vi "invasive_blood_pressure_measurement.vi"() -> ()   [LabVIEW 2020]
uses:
  <vilib>/Math Plots/2D Math Plots/2D Error Bar/2D Error Bar XCtrl/2D Error Bar.xctl
  <vilib>/Utility/file.llb/Write Delimited Spreadsheet (string).vi
  <vilib>/Instr/_visa.llb/VISA Configure Serial Port (Instr).vi
  <vilib>/Utility/file.llb/Write Delimited Spreadsheet (DBL).vi
  <vilib>/Math Plots/2D Math Plots/2D Error Bar/2D Error Bar Datatype/Public/Plot Helper (Fixed).vi
  <vilib>/Analysis/NI_AALBase.lvlib
  <vilib>/Math Plots/2D Math Plots/2D Error Bar/2D Error Bar Datatype/2D Error Bar Datatype.lvclass
  <vilib>/Analysis/NI_AALPro.lvlib
panel:
  out "y":i32
  in  "nule":dbl[](array[numeric])
  out "standard deviation":dbl format="%0.2f"
  out "?":T1(tab)
  in  "?":bool
  in  "baud rate (9600)":u32=9600
  in  "VISA resource name\n(izberi COM1)":refnum<visa-resource-name>
  in  "Stevilo meritev":i32
  in  "Vhodni tlaki [mmHg]":dbl[](array[numeric])
  in  "Shranjevanje podatkov":path
  in  "Cas med meritvami [s]":i32
  in  "Cas med merjenji tlaka [s]":i32
  in  "Referencni tlak [mmHg]":i32
  in  "Shranjevanje podatkov":path
  in  "Stevilo meritev":i32
  in  "Vhodna napetost [V]":i32
  in  "Vhodna napetost [V]":i32
  out "Stanje sistema":string="zacne se meritev"
  out "?":cluster{i32[], dbl[]}(graph)
  out "Povprecna vhodna napetost [V]":dbl
  out "Povprecna izhodna napetost [mV]":dbl
  in  "Prekini merjenje":bool
  out "Velikost tlaka [mmHg]":dbl(slide) scale=0.0..250.0
  out "Izmerjeni tlak [mmHg]":dbl
  out "Konec meritev":string
  out "Poteka merjenje":bool
  in  "Zacni merjenje":bool
  out "Vrednost S [qV/VmmHg]":dbl
  out "Graf vrednosti S":cluster{"napetost":dbl[], "tlak":dbl[]}(graph)
  out "Trenutni vhodni tlak [mmHg]":dbl
  out "Polnjenje tlaka":bool
  out "Zacetna vrednost premice":dbl
  out "Napaka":dbl
  out "?":cluster{i32[], dbl[]}(graph)
  out "Konec meritev":string
  in  "Ustavi merjenje":bool
  in  "Zacni merjenje":bool
  out "Poteka merjenje":bool
  out "Stanje sistema":string="zacne se meritev"
  out "Referencni tlak [mmHg]":dbl(slide) scale=0.0..250.0
  out "Izmerjeni tlak [mmHg]":dbl
  out "Povprecna izhodna napetost [mV]":dbl
  out "Izracunan povprecni\ntlak [mmHg]":dbl
  out "Korekcija tlakov":refnum<class "2D Plot Datatype.lvclass">[](xcontrol) caption="Error Bar Plot"
  in  "Izracunani tlaki [mmHg]":dbl[](array[numeric])
  out "Povprecna vhodna napetost [V]":dbl
  in  "Referencni tlak [mmHg]":dbl[](array[numeric])
  in  "Izhodne (izmerjene)\nnapetosti [mV]":dbl[](array[numeric])
  out "Izmerjeni tlaki [mmHg]":dbl[](array[numeric])
  in  "Korekcija":dbl[](array[numeric])
  out "Vrednost S [qV/VmmHg]":dbl
  in  "Standardna negotovost \nkorekcije u(K)":dbl[](array[numeric])
  # "OSNOVNE NASTAVITVE"
  # "IZVAZIVNO MERJENJE TLAKA"
  # "Invazivna metoda je metoda, ki  neposredno meri arterijski tlak. S pomocjo invazivne metode lahko preprosto belezimo dinamiko krvnega tlaka med posameznimi srcnimi utripi in dolocimo diastolicni in sistolicni krvni tlak. Invazivne metode odlikujejo najvecjo tocnost, ko jo doloca staticna in dinamicna karakteristika pretvornika tlaka."
  # "Dolocitev karakteristike sistema"
  # "Izvajanje meritev tlaka"
  # "UPORABA:\n\n1. Dolocite osnovne nastavitve\n2. Za merjenje karakteristike sistema premaknite veliki gumb levo,\n     za merjenje tlaka pa desno\n3. Vnesite zahtevane vhodne podatke\n         - Dolocitev karakteristike: \n                 * poljubno stevilo vhodnih tlakov, pri katerih se bodo    \n                    izvajale meritve\n                 * stevilo meritev, ki se izvedejo za vsak vhodni tlak\n                 * cas med posameznimi meritvami (v sekundah)\n                 * vhodna napetost, pri kateri se bodo izvajale meritve\n                 * datoteka, v katero se bodo zapisali rezultati\n         - Izvajanje meritev: \n                 * referencni tlak (za izracun merilne negotovosti)\n                 * cas med merjenji (eno merjenje obsega vec meritev, ki \n                    se izvedejo s sekundo zamika)\n                 * stevilo meritev, ki se izvedejo ob vsakem merjenju   \n                   (vsako sekundo)\n                 * vhodna napetost, pri kateri se bodo izvajale meritve\n                 * datoteka, v katero se bodo zapisali rezultati"
  # "MERJENJE TLAKOV"
  # "DOLOCITEV KARAKTERISTIKE SISTEMA"
  # "STANJE MERILNEGA SISTEMA"
  # "PODATKI NAPETOSTI"
  # "PODATKI TLAKA"
  # "REZULTAT MERJENJA KARAKTERISTIKE S"
  # "UPORABA:\n\n1.  Na zacetku SAMO ENKRAT pritisnite gumb \"Zacni \n      merjenje\". \n2.  Ce zelite z merjenjem prenehati, pritisnite gumb \n      \"Prekini merjenje\" (STOP)."
  # "STANJE MERILNEGA SISTEMA"
  # "PODATKI NAPETOSTI"
  # "PODATKI TLAKA"
  # "IZMERJENI TLAKI"
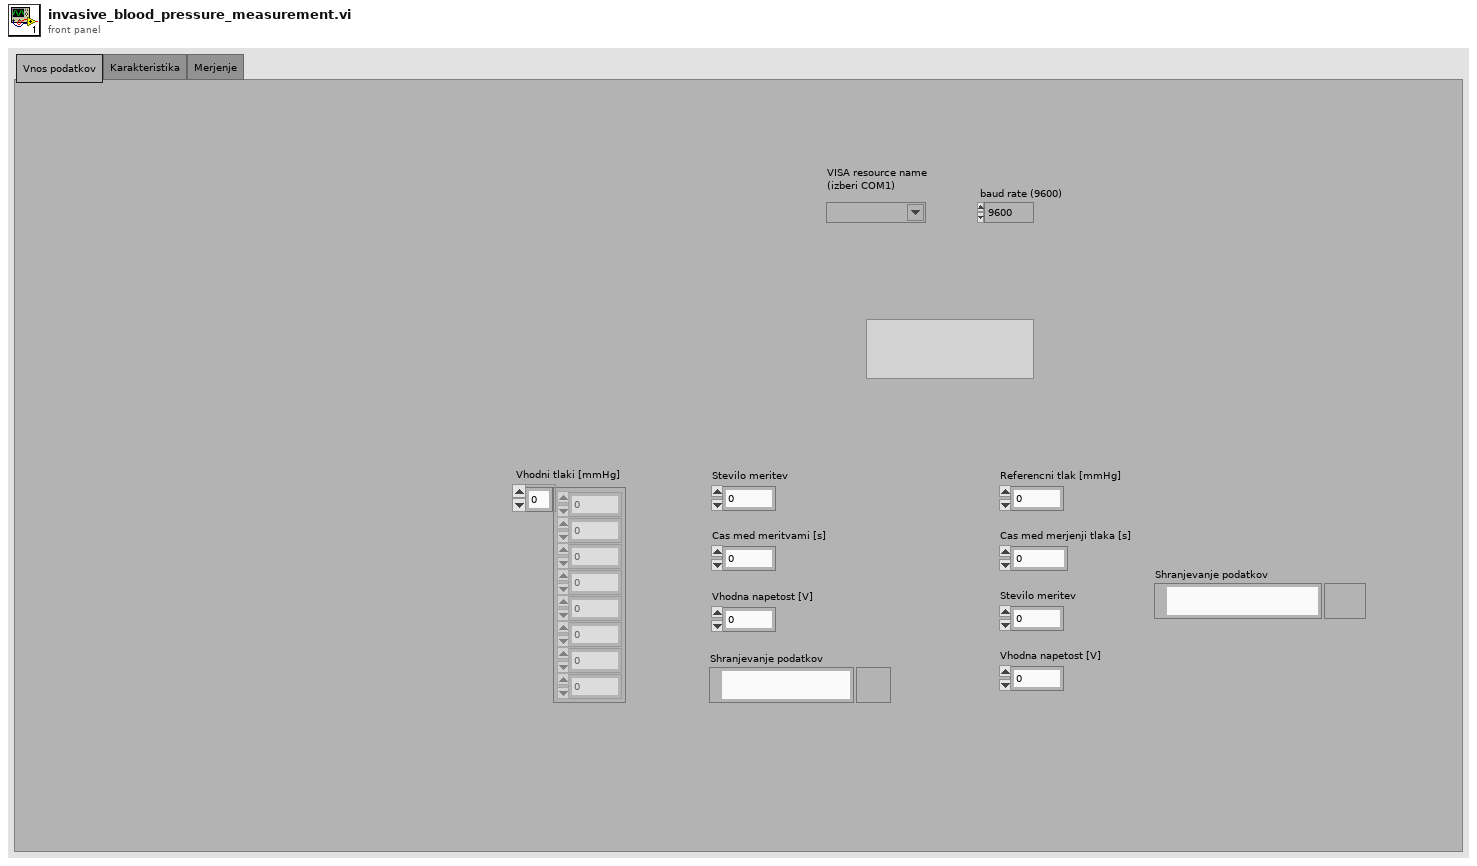
[diagram p1: front panel]
types:
  T1 = enum32{"Vnos podatkov", "Karakteristika", "Merjenje"}
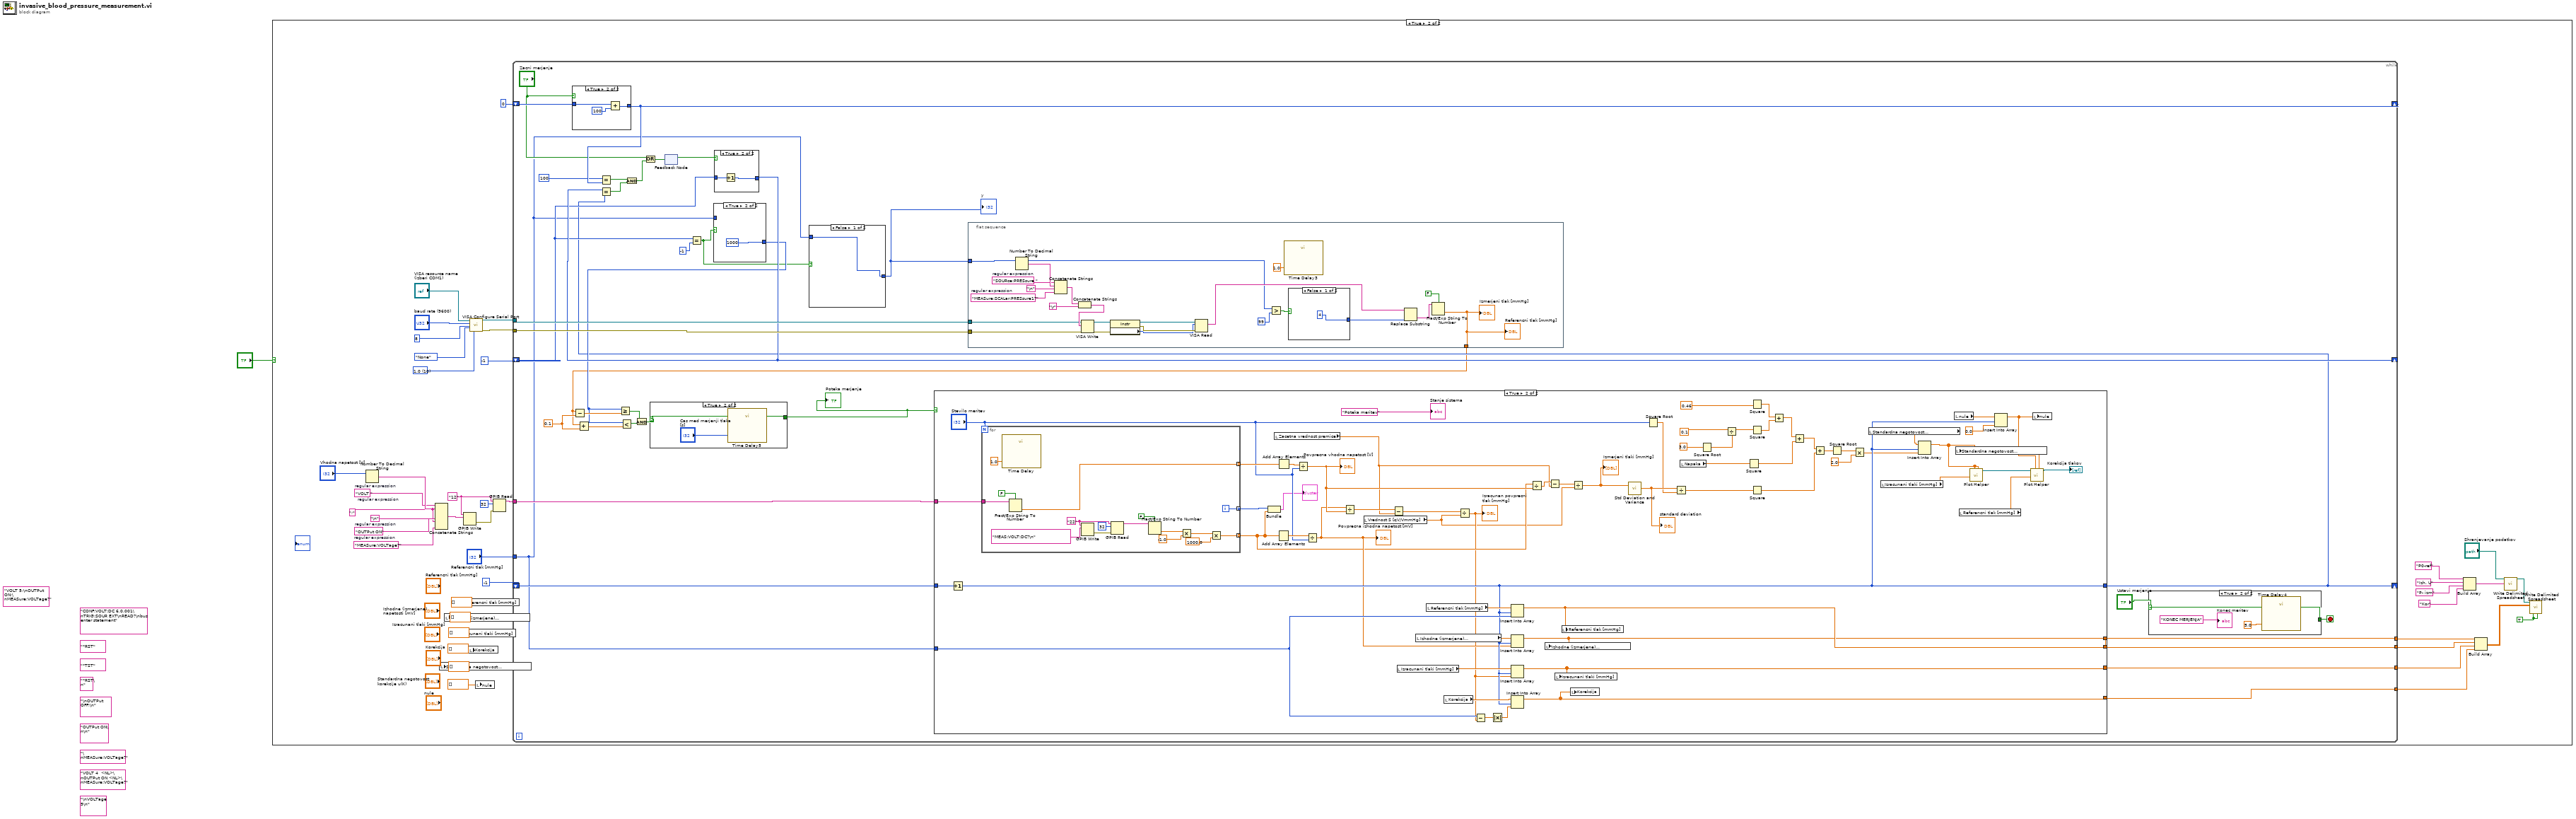
[diagram p0: block diagram]
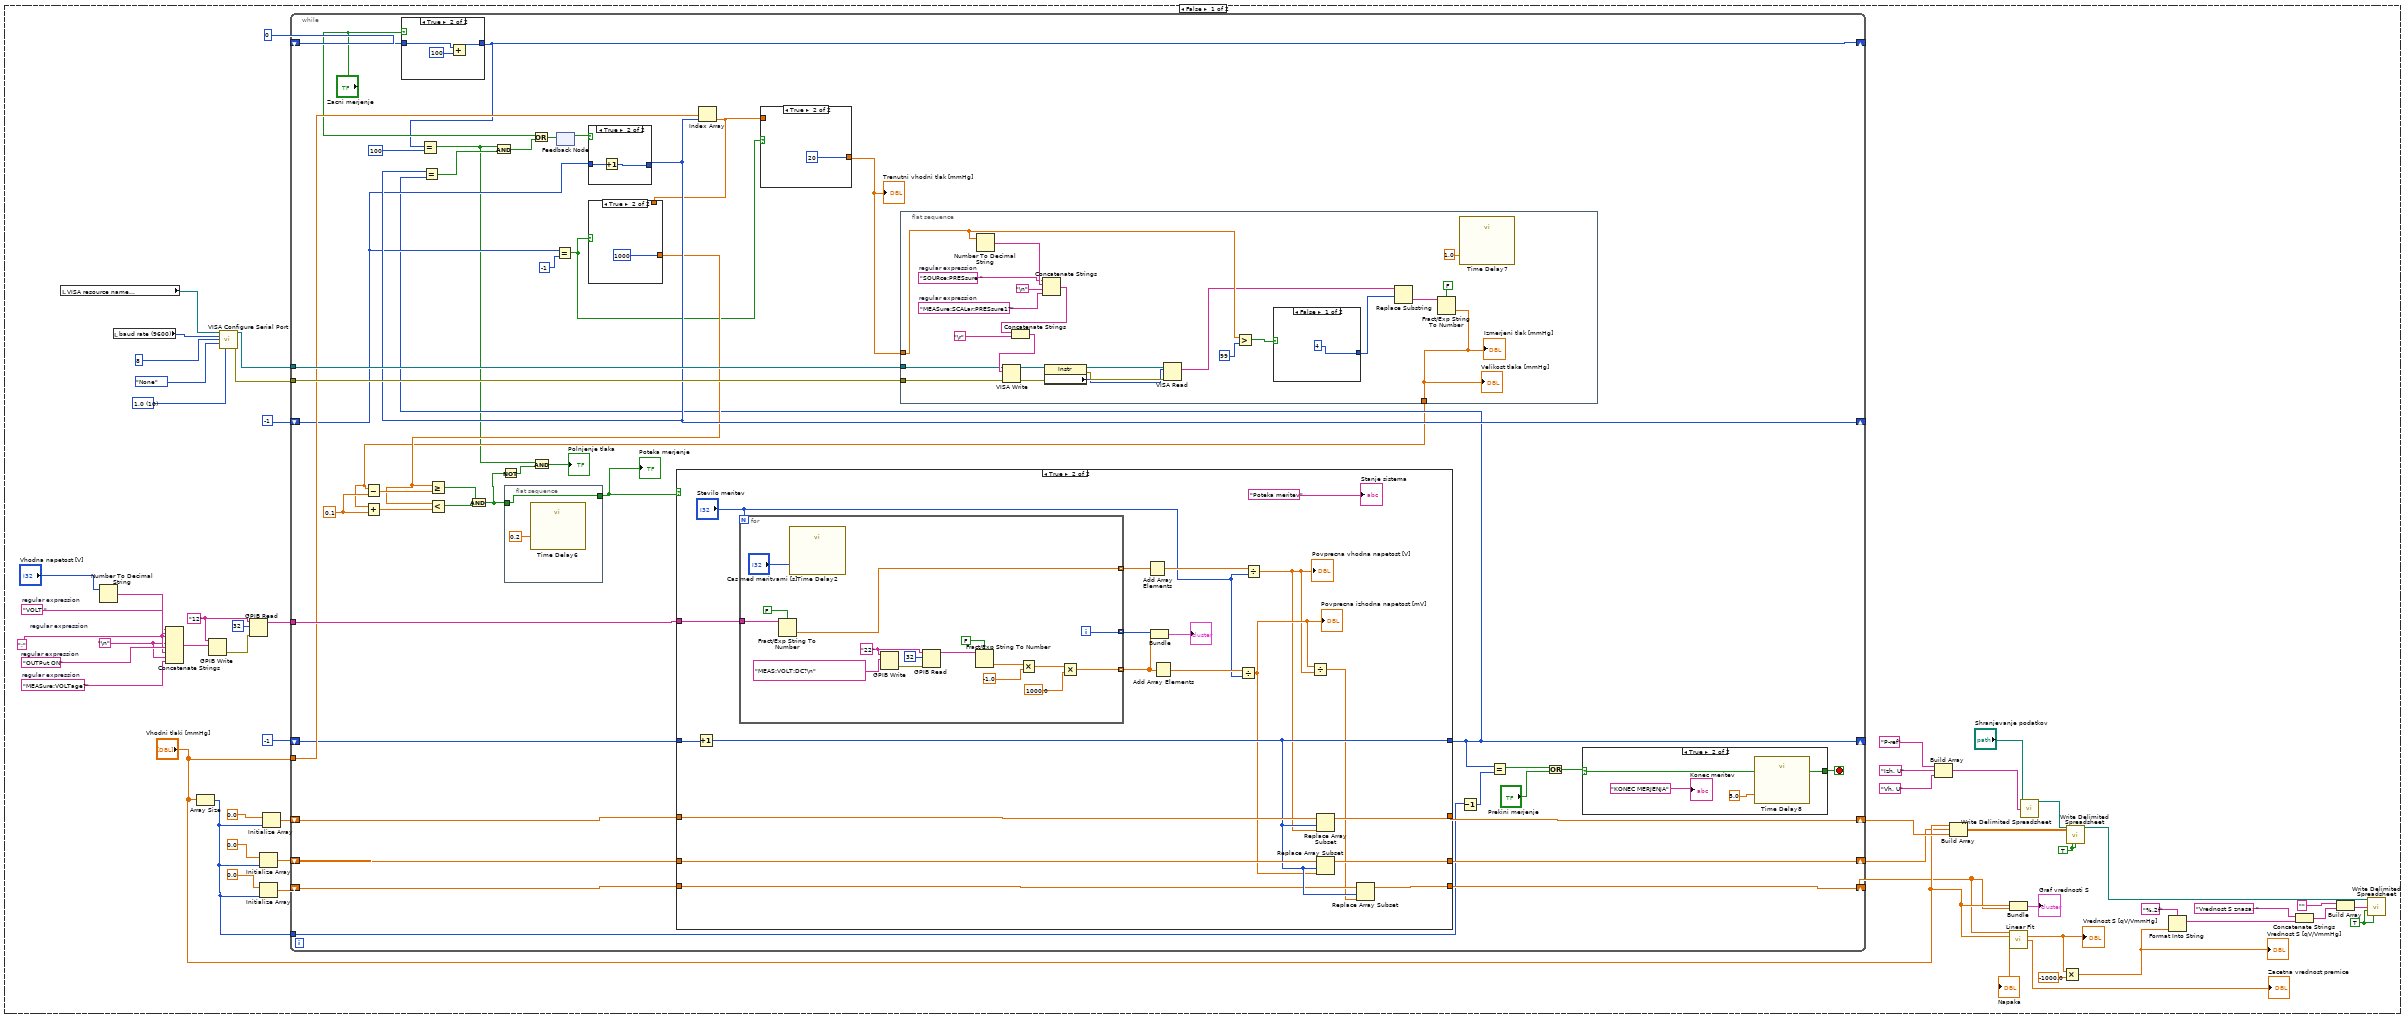
[diagram p2: hidden frame]
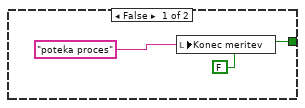
[diagram p4: hidden frame]
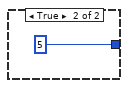
[diagram p8: hidden frame]
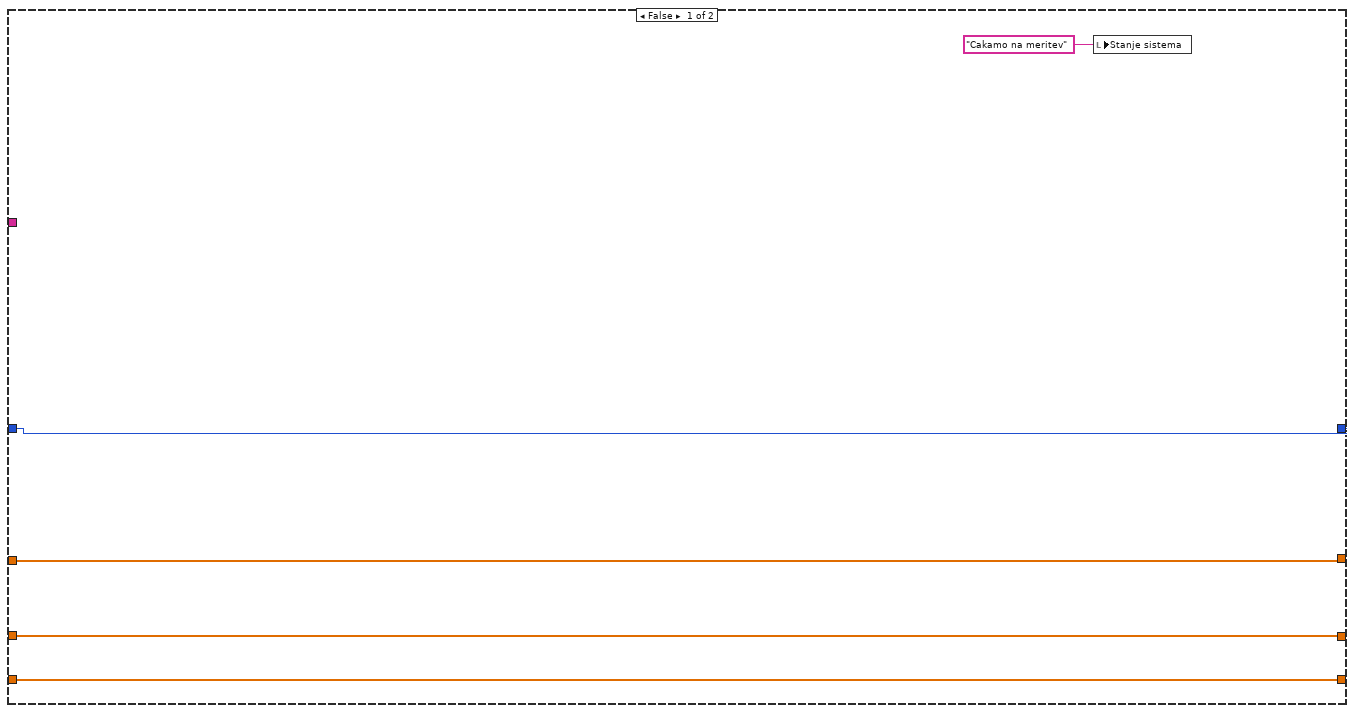
[diagram p9: hidden frame]
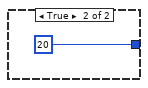
[diagram p10: hidden frame]
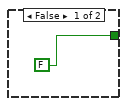
[diagram p11: hidden frame]
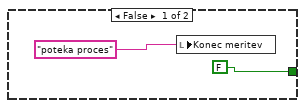
[diagram p12: hidden frame]
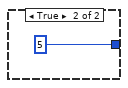
[diagram p16: hidden frame]
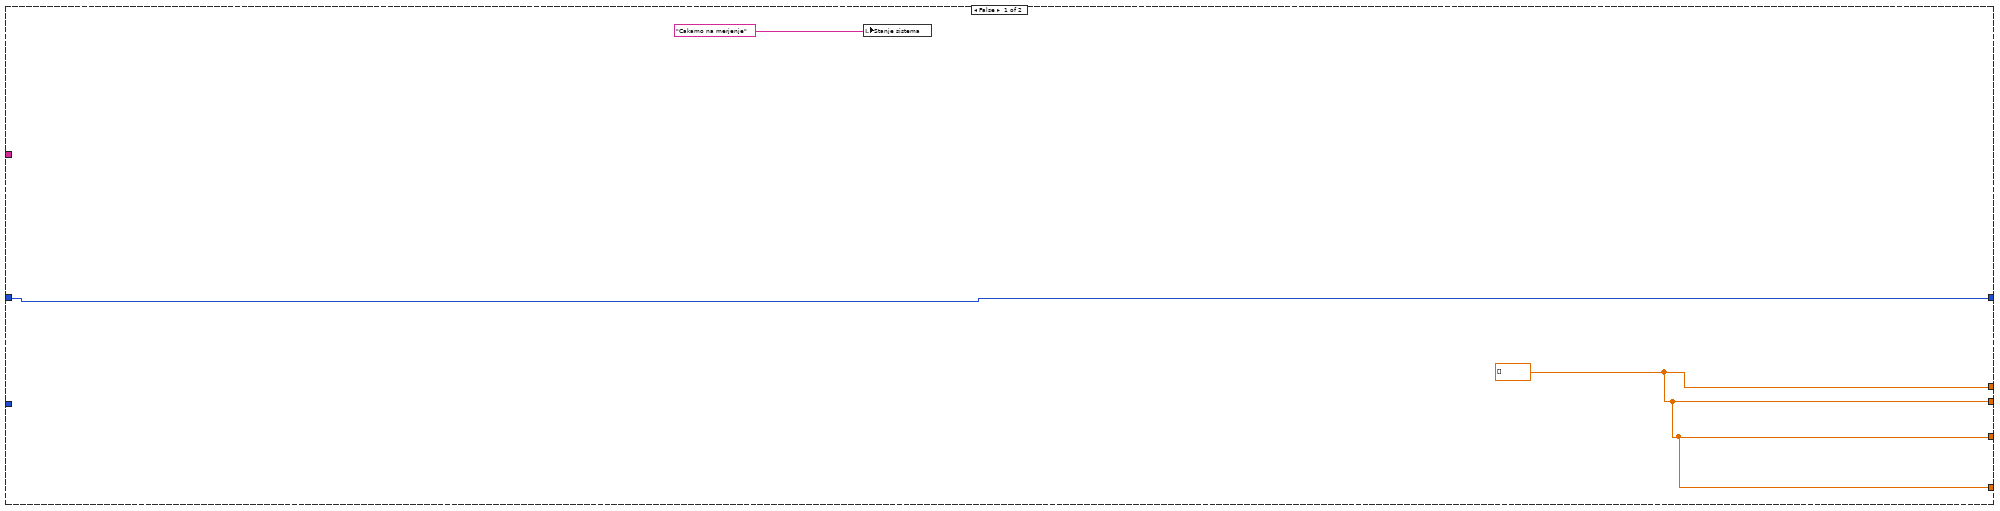
[diagram p17: hidden frame]
diagram:
  (unwired) "VOLT 5;\nOUTPut ON;\nMEASure:VOLTage?" ("data")
  (unwired) "\nOUTPut OFF;\n" ("data")
  (unwired) "\nMEASure:VOLTage?" ("data")
  (unwired) "*TST" ("data")
  (unwired) "*RST" ("data")
  (unwired) "VOLT 4  <NL>\nOUTPut ON <NL>\nMEASure:VOLTage?" ("data")
  (unwired) "\nVOLTage 5\n" ("data")
  (unwired) "*RST\n" ("data")
  (unwired) "CONF:VOLT:DC 6,0.001\nTRIG:SOUR EXT\nREAD?\nbus enter statement" ("data")
  (unwired) "OUTPut ON\n\n" ("data")
  n1 = case shown="True" "?" {
    frame False {
      w16 = u16 10 items=["1.0"=10, "1.5"=15, "2.0"=20] ("stop bits (10: 1 bit)")
      w25 = TRUE ("transpose? (no:F)")
      w32 = "MEASure:VOLTage?"  # regular expression
      w33 = "\n"
      w34 = ";"  # regular expression
      w35 = "OUTPut ON"  # regular expression
      w36 = "VOLT "  # regular expression
      w45 = TRUE ("transpose? (no:F)")
      w55 = "12" ("address string")
      n2 = local read "VISA resource name\n(izberi COM1)"() -> (w3:refnum<visa-resource-name>)
      n3 = Number To Decimal String(number="Vhodna napetost [V]") -> (decimal integer string=w37:string)  [unwired: 1 in]
      n4 = local read "baud rate (9600)"() -> (w4:u32)
      n5 = Concatenate Strings(w36, w37, w34, w33, w35, w34, w33, w32) -> (w29:string)
      n6 = Array Size(array="Vhodni tlaki [mmHg]") -> (size(s)=w11:i32)
      n7 = GPIB Write(0:w55, 1:w29) -> (6:w56:errorcluster)  [unwired: 3 in, 1 out]
      n8 = call-poly "VISA Configure Serial Port"("VISA resource name"=w3, "baud rate (9600)"=w4, "data bits (8)"=u16 8, "parity (0:none)"=enum16{"None", "Odd", "Even", "Mark", "Space"}."None", "stop bits (10: 1 bit)"=w16) -> ("VISA resource name out"=w15:refnum<visa-resource-name>, "error out"=w14:errorcluster)  [unwired: 9 in]
      n9 = GPIB Read(0:w55, 1:32 ("byte count"), 3:w56) -> (5:w53:string)  [unwired: 2 in, 2 out]
      n10 = Initialize Array(0.0 ("new element/subarray"), w11) -> (w40:dbl[])
      n11 = Initialize Array(0.0 ("new element/subarray"), w11) -> (w30:dbl[])
      n12 = Initialize Array(0.0 ("new element/subarray"), w11) -> (w50:dbl[])
      n13 = while {
        tunnel: w53 -> [w100]
        tunnel: "Vhodni tlaki [mmHg]" -> [w90]
        shift-right: [w74] -> _
        shift-left: -1 -> [w81]
        shift-right: [w98] -> w39
        shift-left: w50 -> [w95]
        shift-right: [w97] -> w27
        shift-left: w40 -> [w96]
        shift-right: [w93] -> w19
        shift-left: w30 -> [w94]
        tunnel: w15 -> [w92]
        tunnel: w14 -> [w91]
        shift-right: [w80] -> _
        shift-left: -1 -> [w76]
        shift-right: [w58] -> _
        shift-left: 0 -> [w85]
        tunnel: w11 -> [w73]
        stop <- w68 stop-if-true
        w89 = 0.1 ("y")
        n14 = Subtract(x=w67, y=w89) -> (x-y=w87:dbl)
        n15 = Add(x=w67, y=w89) -> (x+y=w88:dbl)
        n16 = case shown="True" "Zacni merjenje" {
          tunnel: w85 -> [w110 w113]
          tunnel: [w110 w111] -> w58
          frame False {
          }
          frame True {
            n17 = Add(x=w113, y=100) -> (x+y=w111:i32)
          }
        }
        n18 = Equal?(x=w58, y=100 ("x")) -> (x = y?=w62:bool)
        n19 = flat-sequence {
          tunnel: w61 -> [w142]
          tunnel: [w142] -> w99
          frame #0 {
            n20 = call "Time Delay6"("Delay Time (s)"=0.2) -> ()  [unwired: 10 in, 1 out]
          }
        }
        n21 = Equal?(x=w76, y=-1) -> (x = y?=w66:bool)
        n22 = feedback #1() -> (w82:bool)  [unwired: 1 in]
        n23 = case shown="True" w82 {
          tunnel: w76 -> [w114 w116]
          tunnel: [w114 w115] -> w80
          frame False {
          }
          frame True {
            n24 = Increment(x=w116) -> (x+1=w115:i32)
          }
        }
        n25 = case shown="True" w99 {
          tunnel: w100 -> [_ w161]
          tunnel: [w144 w160] -> w98
          tunnel: [w147 w159] -> w97
          tunnel: w96 -> [w147 w158]
          tunnel: w95 -> [w144 w157]
          tunnel: w81 -> [w148 w156]
          tunnel: [w148 w154] -> w74
          tunnel: w94 -> [w145 w153]
          tunnel: [w145 w152] -> w93
          frame False {
            n26 = local write "Stanje sistema"("Cakamo na meritev") -> ()
          }
          frame True {
            n27 = Increment(x=w156) -> (x+1=w154:i32)
            n28 = for {
              N: "Stevilo meritev" -> [_]
              tunnel: [w173] -> w163 mode=indexing
              tunnel: [w172] -> w167 mode=indexing
              tunnel: [w171] -> w164 mode=indexing
              tunnel: w161 -> [w170]
              i -> [w171]
              w184 = "22" ("address string")
              n29 = Fract/Exp String To Number(use system decimal point (T)=FALSE, string=w170) -> (number=w172:dbl)  [unwired: 2 in, 1 out]
              n30 = call "Time Delay2"("Delay Time (s)"="Cas med meritvami [s]") -> ()  [unwired: 10 in, 1 out]
              n31 = GPIB Write(0:w184, 1:"MEAS:VOLT:DC?\n" ("data")) -> (6:w182:errorcluster)  [unwired: 3 in, 1 out]
              n32 = GPIB Read(0:w184, 1:32 ("byte count"), 3:w182) -> (5:w176:string)  [unwired: 2 in, 2 out]
              n33 = Fract/Exp String To Number(use system decimal point (T)=FALSE, string=w176) -> (number=w180:dbl)  [unwired: 2 in, 1 out]
              n34 = Multiply(x=w180, y=-1.0) -> (x*y=w175:dbl)
              n35 = Multiply(x=w175, y=1000.0) -> (x*y=w173:dbl)
            }
            n36 = Add Array Elements(numeric array=w167) -> (sum=w166:dbl)
            n37 = Bundle(w164, w163) -> (→"?":cluster{i32[], dbl[]})  [unwired: 1 in]
            n38 = Add Array Elements(numeric array=w163) -> (sum=w168:dbl)
            n39 = Divide(x=w168, y="Stevilo meritev") -> (x/y=w151:dbl)
            "Povprecna izhodna napetost [mV]" <- w151
            n40 = Divide(x=w166, y="Stevilo meritev") -> (x/y=w150:dbl)
            "Povprecna vhodna napetost [V]" <- w150
            n41 = Divide(x=w151, y=w150) -> (x/y=w149:dbl)
            n42 = Replace Array Subset(array=w157, new element=w150, index=w154) -> (w160:dbl[])
            n43 = Replace Array Subset(array=w158, new element=w151, index=w154) -> (w159:dbl[])
            n44 = Replace Array Subset(array=w153, new element=w149, index=w154) -> (w152:dbl[])
            "Stanje sistema" <- "Poteka meritev"
          }
        }
        n45 = Equal?(x=w80, y=w74) -> (x = y?=w79:bool)
        n46 = And(x=w62, y=w79) -> (x .and. y?=w78:bool)
        n47 = Or(x="Zacni merjenje", y=w78) -> (x .or. y?=w83:bool)
        n48 = feedback-in #1(w83) -> ()
        n49 = Index Array(array=w90, index=w80) -> (element=w64:dbl)
        n50 = case shown="True" w66 {
          tunnel: [w108 1000 ("y")] -> w75
          tunnel: w64 -> [w108 _]
          frame False {
          }
          frame True {
          }
        }
        n51 = Greater Or Equal?(x=w75, y=w87) -> (x >= y?=w63:bool)
        n52 = Less?(x=w75, y=w88) -> (x < y?=w86:bool)
        n53 = And(x=w63, y=w86) -> (x .and. y?=w61:bool)
        n54 = Not(x=w61) -> (.not. x?=w60:bool)
        n55 = And(x=w62, y=w60) -> (x .and. y?=→"Polnjenje tlaka":bool)
        n56 = case shown="True" w66 {
          tunnel: [w101 20 ("y")] -> w65
          tunnel: w64 -> [w101 _]
          frame False {
          }
          frame True {
          }
        }
        "Trenutni vhodni tlak [mmHg]" <- w65
        n57 = flat-sequence {
          tunnel: w92 -> [w127]
          tunnel: w91 -> [w126]
          tunnel: w65 -> [w119]
          tunnel: [w117] -> w67
          frame #0 {
            w129 = "MEASure:SCALar:PRESsure1?"  # regular expression
            w131 = "SOURce:PRESsure "  # regular expression
            n58 = Number To Decimal String(number=w119) -> (decimal integer string=w132:string)  [unwired: 1 in]
            n59 = Concatenate Strings(w131, w132, "\n", w129) -> (w128:string)
            n60 = Concatenate Strings(w128, "\r") -> (w133:string)
            n61 = VISA Write(VISA resource name=w127, write buffer=w133, error in (no error)=w126) -> (VISA resource name out=w139:refnum<visa-resource-name>, error out=w136:errorcluster)  [unwired: 1 out]
            n62 = property class="Instr"(reference=w139, error in=w136) -> (reference out=w138:refnum<visa-resource-name>, error out=w137:errorcluster, "Serial Settings:Number of Bytes at Serial Port"=w135:u32)
            n63 = VISA Read(VISA resource name=w138, byte count=w135, error in (no error)=w137) -> (read buffer=w118:string)  [unwired: 3 out]
            n64 = Greater?(x=w119, y=99) -> (0:w123:bool)
            n65 = case shown="False" w123 {
              tunnel: [4 ("y") 5 ("y")] -> w122
              frame False {
              }
              frame True {
              }
            }
            n66 = Replace Substring(2:w122, 5:w118) -> (0:w121:string)  [unwired: 2 in, 1 out]
            n67 = Fract/Exp String To Number(use system decimal point (T)=FALSE, string=w121) -> (number=w117:dbl)  [unwired: 2 in, 1 out]
            "Izmerjeni tlak [mmHg]" <- w117
            "Velikost tlaka [mmHg]" <- w117
            n68 = call "Time Delay7"("Delay Time (s)"=1.0) -> ()  [unwired: 10 in, 1 out]
          }
        }
        n69 = Decrement(x=w73) -> (x-1=w72:i32)
        n70 = Equal?(x=w74, y=w72) -> (x = y?=w70:bool)
        n71 = Or(x=w70, y="Prekini merjenje") -> (x .or. y?=w69:bool)
        n72 = case shown="True" w69 {
          selector: w69 -> [_ w105]
          tunnel: [FALSE w105] -> w68
          frame False {
            n73 = local write "Konec meritev"("poteka proces") -> ()
          }
          frame True {
            n74 = call "Time Delay8"("Delay Time (s)"=5.0) -> ()  [unwired: 10 in, 1 out]
            "Konec meritev" <- "KONEC MERJENJA"
          }
        }
        "Poteka merjenje" <- w99
      }
      n75 = Build Array("P-ref", "Izh. U", "Vh. U") -> (w47:string[])
      n76 = Build Array("Vhodni tlaki [mmHg]", w27, w39) -> (w43:dbl[][])
      n77 = Bundle("Vhodni tlaki [mmHg]"="Vhodni tlaki [mmHg]", w19) -> (→"Graf vrednosti S":cluster{" Vhodni tlaki [mmHg]":dbl[], dbl[]})  [unwired: 1 in]
      n78 = call <vilib>:"Linear Fit.vi"("Y"=w19, "X"="Vhodni tlaki [mmHg]") -> ("slope"=w8:dbl, "intercept"=→"Zacetna vrednost premice":dbl, "residue"=→"Napaka":dbl)  [unwired: 9 in, 2 out]
      "Vrednost S [qV/VmmHg]" <- w8
      n79 = call-poly <vilib>:"Write Delimited Spreadsheet.vi"("file path (dialog if empty)"="Shranjevanje podatkov", "1D data"=w47) -> ("new file path (Not A Path if cancelled)"=w46:path)  [unwired: 12 in, 1 out]
      n80 = Multiply(x=w8, y=-1000.0) -> (x*y=w6:dbl)
      "Vrednost S [qV/VmmHg]" <- w6
      n81 = call-poly <vilib>:"Write Delimited Spreadsheet.vi"("file path (dialog if empty)"=w46, "2D data"=w43, "append to file? (new file:F)"=w45, "transpose? (no:F)"=w45) -> ("new file path (Not A Path if cancelled)"=w20:path)  [unwired: 10 in, 1 out]
      n82 = Format Into String(format string="%.2f", w6) -> (resulting string=w7:string)  [unwired: 2 in, 1 out]
      n83 = Concatenate Strings("Vrednost S znasa: ", w7) -> (w21:string)
      n84 = Build Array("", w21) -> (w24:string[])
      n85 = call-poly <vilib>:"Write Delimited Spreadsheet.vi"("file path (dialog if empty)"=w20, "1D data"=w24, "append to file? (new file:F)"=w25, "transpose? (no:F)"=w25) -> ()  [unwired: 10 in, 2 out]
    }
    frame True {
      w202 = u16 10 items=["1.0"=10, "1.5"=15, "2.0"=20] ("stop bits (10: 1 bit)")
      w208 = "MEASure:VOLTage?"  # regular expression
      w209 = "\n"
      w210 = ";"  # regular expression
      w211 = "OUTPut ON"  # regular expression
      w212 = "VOLT "  # regular expression
      w217 = TRUE ("transpose? (no:F)")
      w225 = "12" ("address string")
      n86 = Number To Decimal String(number="Vhodna napetost [V]") -> (decimal integer string=w213:string)  [unwired: 1 in]
      n87 = Concatenate Strings(w212, w213, w210, w209, w211, w210, w209, w208) -> (w207:string)
      n88 = local write "Standardna negotovost \nkorekcije u(K)"(dbl[] []) -> ()
      n89 = local write "Izhodne (izmerjene)\nnapetosti [mV]"(dbl[] []) -> ()
      n90 = local write "Izracunani tlaki [mmHg]"(dbl[] []) -> ()
      n91 = local write "Referencni tlak [mmHg]"(dbl[] []) -> ()
      n92 = GPIB Write(0:w225, 1:w207) -> (6:w226:errorcluster)  [unwired: 3 in, 1 out]
      n93 = local write "Korekcija"(dbl[] []) -> ()
      n94 = call-poly "VISA Configure Serial Port"("VISA resource name"="VISA resource name\n(izberi COM1)", "baud rate (9600)"="baud rate (9600)", "data bits (8)"=u16 8, "parity (0:none)"=enum16{"None", "Odd", "Even", "Mark", "Space"}."None", "stop bits (10: 1 bit)"=w202) -> ("VISA resource name out"=w201:refnum<visa-resource-name>, "error out"=w200:errorcluster)  [unwired: 9 in]
      n95 = local write "nule"(dbl[] []) -> ()
      n96 = GPIB Read(0:w225, 1:32 ("byte count"), 3:w226) -> (5:w223:string)  [unwired: 2 in, 2 out]
      n97 = while {
        tunnel: w223 -> [w261]
        shift-right: [w240] -> _
        shift-left: -1 -> [w248]
        tunnel: w201 -> [w260]
        tunnel: w200 -> [w259]
        shift-right: [w246] -> _
        shift-left: -1 -> [w242]
        shift-right: [w253] -> _
        shift-left: 0 -> [w254]
        tunnel: "Referencni tlak [mmHg]" -> [w234]
        tunnel: [w230] -> w188
        tunnel: [w229] -> w187
        tunnel: [w228] -> w186
        tunnel: [w227] -> w185
        stop <- w239 stop-if-true
        w238 = 0.1 ("y")
        n98 = case shown="True" "Zacni merjenje" {
          tunnel: w254 -> [w274 w277]
          tunnel: [w274 w275] -> w253
          frame False {
          }
          frame True {
            n99 = Add(x=w277, y=100) -> (x+y=w275:i32)
          }
        }
        n100 = Subtract(x=w235, y=w238) -> (x-y=w257:dbl)
        n101 = Add(x=w235, y=w238) -> (x+y=w258:dbl)
        n102 = Equal?(x=100, y=w253) -> (x = y?=w247:bool)
        n103 = feedback #2() -> (w249:bool)  [unwired: 1 in]
        n104 = Equal?(x=w242, y=-1) -> (x = y?=w232:bool)
        n105 = case shown="True" w232 {
          tunnel: [w272 1000 ("y")] -> w241
          tunnel: w234 -> [w272 _]
          frame False {
          }
          frame True {
          }
        }
        n106 = Greater Or Equal?(x=w241, y=w257) -> (x >= y?=w256:bool)
        n107 = Less?(x=w241, y=w258) -> (x < y?=w255:bool)
        n108 = And(x=w256, y=w255) -> (x .and. y?=w237:bool)
        n109 = case shown="True" w237 {
          selector: w237 -> [_ w266]
          tunnel: [FALSE w266] -> w231
          frame False {
          }
          frame True {
            n110 = call "Time Delay5"("Delay Time (s)"="Cas med merjenji tlaka [s]") -> ()  [unwired: 10 in, 1 out]
          }
        }
        "Poteka merjenje" <- w231
        n111 = case shown="True" w249 {
          tunnel: w242 -> [w278 w280]
          tunnel: [w278 w279] -> w246
          frame False {
          }
          frame True {
            n112 = Increment(x=w280) -> (x+1=w279:i32)
          }
        }
        n113 = case shown="False" w232 {
          tunnel: [w262 20 ("y")] -> w233
          tunnel: w234 -> [w262 _]
          frame False {
          }
          frame True {
          }
        }
        "y" <- w233
        n114 = case shown="True" w231 {
          tunnel: w261 -> [_ w364]
          tunnel: w248 -> [w308 w363]
          tunnel: [w308 w340] -> w240
          tunnel: w234 -> [_ w347]
          tunnel: [w306 w339] -> w230
          tunnel: [w306 w338] -> w229
          tunnel: [w306 w337] -> w228
          tunnel: [w306 w336] -> w227
          frame False {
            w306 = dbl[] []
            n115 = local write "Stanje sistema"("Cakamo na merjenje") -> ()
          }
          frame True {
            n116 = Increment(x=w363) -> (x+1=w340:i32)
            n117 = for {
              N: "Stevilo meritev" -> [_]
              tunnel: [w372] -> w319 mode=indexing
              tunnel: [w371] -> w367 mode=indexing
              tunnel: [w370] -> w365 mode=indexing
              tunnel: w364 -> [w369]
              i -> [w370]
              w384 = "22" ("address string")
              n118 = call "Time Delay"("Delay Time (s)"=1.0) -> ()  [unwired: 10 in, 1 out]
              n119 = Fract/Exp String To Number(use system decimal point (T)=FALSE, string=w369) -> (number=w371:dbl)  [unwired: 2 in, 1 out]
              n120 = GPIB Write(0:w384, 1:"MEAS:VOLT:DC?\n" ("data")) -> (6:w382:errorcluster)  [unwired: 3 in, 1 out]
              n121 = GPIB Read(0:w384, 1:32 ("byte count"), 3:w382) -> (5:w375:string)  [unwired: 2 in, 2 out]
              n122 = Fract/Exp String To Number(use system decimal point (T)=FALSE, string=w375) -> (number=w379:dbl)  [unwired: 2 in, 1 out]
              n123 = Multiply(x=w379, y=-1.0) -> (x*y=w374:dbl)
              n124 = Multiply(x=w374, y=1000.0) -> (x*y=w372:dbl)
            }
            n125 = Bundle(w365, w319) -> (→"?":cluster{i32[], dbl[]})  [unwired: 1 in]
            n126 = local read "Zacetna vrednost premice"() -> (w311:dbl)
            n127 = Add Array Elements(numeric array=w319) -> (sum=w368:dbl)
            n128 = Add Array Elements(numeric array=w367) -> (sum=w366:dbl)
            n129 = Divide(x=w366, y="Stevilo meritev") -> (x/y=w352:dbl)
            "Povprecna vhodna napetost [V]" <- w352
            n130 = Divide(x=w368, y="Stevilo meritev") -> (x/y=w320:dbl)
            "Povprecna izhodna napetost [mV]" <- w320
            n131 = Divide(x=w320, y=w352) -> (x/y=w313:dbl)
            n132 = local read "Vrednost S [qV/VmmHg]"() -> (w315:dbl)
            n133 = Subtract(x=w313, y=w311) -> (x-y=w318:dbl)
            n134 = local read "Izracunani tlaki [mmHg]"() -> (w349:dbl[])
            n135 = local read "Izhodne (izmerjene)\nnapetosti [mV]"() -> (w346:dbl[])
            n136 = local read "Referencni tlak [mmHg]"() -> (w348:dbl[])
            n137 = local read "Korekcija"() -> (w351:dbl[])
            n138 = Divide(x=w318, y=w315) -> (x/y=w317:dbl)
            "Izracunan povprecni\ntlak [mmHg]" <- w317
            n139 = Subtract(x=w347, y=w317) -> (x-y=w361:dbl)
            n140 = Absolute Value(x=w361) -> (abs(x)=w350:dbl)
            n141 = Insert Into Array(array=w348, index=w340, new element=w347) -> (w339:dbl[])
            n142 = Insert Into Array(array=w346, index=w340, new element=w320) -> (w338:dbl[])
            n143 = Insert Into Array(array=w349, index=w340, new element=w317) -> (w337:dbl[])
            n144 = Insert Into Array(array=w351, index=w340, new element=w350) -> (w336:dbl[])
            n145 = Divide(x=w319, y=w352) -> (x/y=w312:dbl[])
            n146 = local write "Izhodne (izmerjene)\nnapetosti [mV]"(w338) -> ()
            n147 = Subtract(x=w312, y=w311) -> (x-y=w316:dbl[])
            n148 = local write "Izracunani tlaki [mmHg]"(w337) -> ()
            n149 = local write "Referencni tlak [mmHg]"(w339) -> ()
            n150 = local write "Korekcija"(w336) -> ()
            n151 = Divide(x=w316, y=w315) -> (x/y=w314:dbl[])
            "Izmerjeni tlaki [mmHg]" <- w314
            n152 = call <vilib>:"Std Deviation and Variance.vi"("X"=w314) -> ("standard deviation"=w359:dbl)  [unwired: 1 in, 2 out]
            "standard deviation" <- w359
            n153 = Square Root(x="Stevilo meritev") -> (sqrt(x)=w358:dbl)
            n154 = Divide(x=w359, y=w358) -> (x/y=w327:dbl)
            n155 = local read "Napaka"() -> (w309:dbl)
            n156 = Square Root(x=3.0) -> (sqrt(x)=w331:dbl)
            n157 = Divide(x=0.1, y=w331) -> (x/y=w329:dbl)
            n158 = Square(x=w309) -> (x^2=w333:dbl)
            n159 = Square(x=0.46) -> (x^2=w335:dbl)
            n160 = Square(x=w329) -> (x^2=w332:dbl)
            n161 = Square(x=w327) -> (x^2=w326:dbl)
            n162 = Add(x=w335, y=w332) -> (x+y=w334:dbl)
            n163 = Add(x=w334, y=w333) -> (x+y=w325:dbl)
            n164 = Add(x=w325, y=w326) -> (x+y=w324:dbl)
            n165 = Square Root(x=w324) -> (sqrt(x)=w322:dbl)
            n166 = Multiply(x=w322, y=2.0) -> (x*y=w321:dbl)
            n167 = local read "Standardna negotovost \nkorekcije u(K)"() -> (w342:dbl[])
            n168 = local read "Izracunani tlaki [mmHg]"() -> (w357:dbl[])
            n169 = Insert Into Array(array=w342, index=w340, new element=w321) -> (w341:dbl[])
            n170 = local read "nule"() -> (w344:dbl[])
            n171 = local write "Standardna negotovost \nkorekcije u(K)"(w341) -> ()
            n172 = local read "Referencni tlak [mmHg]"() -> (w354:dbl[])
            n173 = call-poly <vilib>:"Plot Helper.vi"("error b vector"=w341, "error a vector"=w341, "y vector"=w357) -> ("2D Plot Class Obj Array out"=w356:refnum<class "2D Plot Datatype.lvclass">[])  [unwired: 3 in, 5 out]
            n174 = Insert Into Array(array=w344, index=w340, new element=0.0 ("new element/subarray")) -> (w343:dbl[])
            n175 = call-poly <vilib>:"Plot Helper.vi"("error b vector"=w343, "error a vector"=w343, "y vector"=w354, "2D Plot Class Obj Array in"=w356) -> ("2D Plot Class Obj Array out"=→"Korekcija tlakov":refnum<class "2D Plot Datatype.lvclass">[])  [unwired: 2 in, 5 out]
            n176 = local write "nule"(w343) -> ()
            "Stanje sistema" <- "Poteka meritev"
          }
        }
        n177 = Equal?(x=w246, y=w240) -> (x = y?=w245:bool)
        n178 = And(x=w247, y=w245) -> (x .and. y?=w244:bool)
        n179 = Or(x="Zacni merjenje", y=w244) -> (x .or. y?=w250:bool)
        n180 = feedback-in #2(w250) -> ()
        n181 = flat-sequence {
          tunnel: w260 -> [w291]
          tunnel: w259 -> [w290]
          tunnel: w233 -> [w281]
          tunnel: [w282] -> w235
          frame #0 {
            w293 = "MEASure:SCALar:PRESsure1?"  # regular expression
            w295 = "SOURce:PRESsure "  # regular expression
            n182 = Number To Decimal String(number=w281) -> (decimal integer string=w296:string)  [unwired: 1 in]
            n183 = Concatenate Strings(w295, w296, "\n", w293) -> (w292:string)
            n184 = Concatenate Strings(w292, "\r") -> (w297:string)
            n185 = VISA Write(VISA resource name=w291, write buffer=w297, error in (no error)=w290) -> (VISA resource name out=w303:refnum<visa-resource-name>, error out=w300:errorcluster)  [unwired: 1 out]
            n186 = property class="Instr"(reference=w303, error in=w300) -> (reference out=w302:refnum<visa-resource-name>, error out=w301:errorcluster, "Serial Settings:Number of Bytes at Serial Port"=w299:u32)
            n187 = VISA Read(VISA resource name=w302, byte count=w299, error in (no error)=w301) -> (read buffer=w283:string)  [unwired: 3 out]
            n188 = Greater?(x=w281, y=99) -> (0:w287:bool)
            n189 = call "Time Delay3"("Delay Time (s)"=1.0) -> ()  [unwired: 10 in, 1 out]
            n190 = case shown="False" w287 {
              tunnel: [4 ("y") 5 ("y")] -> w286
              frame False {
              }
              frame True {
              }
            }
            n191 = Replace Substring(2:w286, 5:w283) -> (0:w285:string)  [unwired: 2 in, 1 out]
            n192 = Fract/Exp String To Number(use system decimal point (T)=FALSE, string=w285) -> (number=w282:dbl)  [unwired: 2 in, 1 out]
            "Izmerjeni tlak [mmHg]" <- w282
            "Referencni tlak [mmHg]" <- w282
          }
        }
        n193 = case shown="True" "Ustavi merjenje" {
          selector: "Ustavi merjenje" -> [_ w269]
          tunnel: [FALSE w269] -> w239
          frame False {
            n194 = local write "Konec meritev"("poteka proces") -> ()
          }
          frame True {
            n195 = call "Time Delay4"("Delay Time (s)"=5.0) -> ()  [unwired: 10 in, 1 out]
            "Konec meritev" <- "KONEC MERJENJA"
          }
        }
      }
      n196 = Build Array("P0-ref", "Izh. U", "P- izm", "Kor") -> (w219:string[])
      n197 = Build Array(w188, w187, w186, w185) -> (w192:dbl[][])
      n198 = call-poly <vilib>:"Write Delimited Spreadsheet.vi"("file path (dialog if empty)"="Shranjevanje podatkov", "1D data"=w219) -> ("new file path (Not A Path if cancelled)"=w218:path)  [unwired: 12 in, 1 out]
      n199 = call-poly <vilib>:"Write Delimited Spreadsheet.vi"("file path (dialog if empty)"=w218, "2D data"=w192, "append to file? (new file:F)"=w217, "transpose? (no:F)"=w217) -> ()  [unwired: 10 in, 2 out]
    }
  }
